vi "rs3 init devices_and_sensors.vi"(6 "rscontext":u64=1752067024, 8 "error in":errorcluster, 9 "api_version":i32=20710, 10 "Select Device":i32, 11 "Select Sensor":i32) -> (0 "error out":errorcluster, 1 "Adv. enable?":i32, 2 "init results":T3, 3 "init error":string, 4 "All Devices":T2(array[cluster]), 5 "Sensor Array":T1(array[cluster]), 7 "Found RealSense":bool)   [LabVIEW 2019, in "libRealSense3.lvlib"]
doc: "Initialized the RealSense device. \nSelect the specific DEVICE and its specific SENSOR. \n\n\nINPUT:\nSelect Device The INDEX to the specific DEVICE handle\nSelect Sensor The INDEX to the specific SENSOR that is part of the selected DEVICE.\n \nOUTPUT:\ninit result Contains all the information about the selected device and its sensor. You will need to use the Dev Out HANDLE to communicate with the device. \n \nselected sensor array Contains the arrays of SENSORS attached to a specific DEVICE.\nall devices Contains array of all device that are attached to the PC."
uses:
  libRealSense3.lvlib
panel:
  # "RS3 Init Device and Sensors"
  # "(C) Intel Corp. 2017,  AGJ"
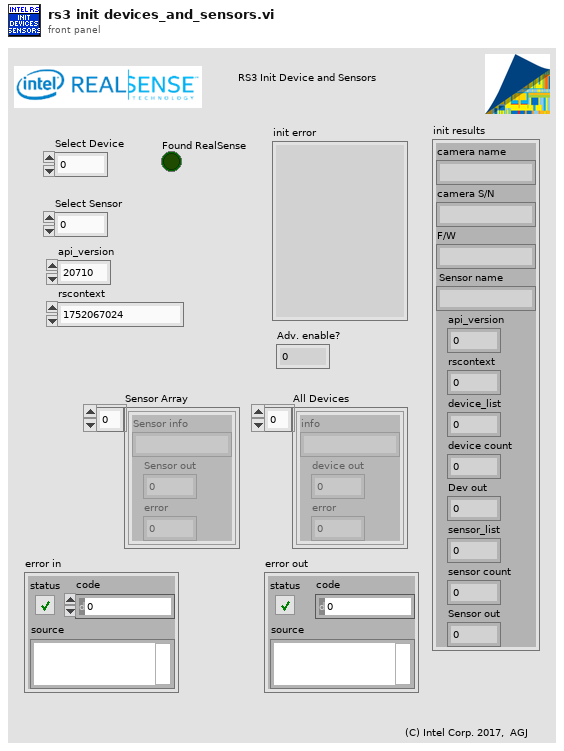
[diagram p1: front panel]
types:
  T1 = cluster{"Sensor info":string, "Sensor out":u64, "error":u64}[]
  T2 = cluster{"info":string, "device out":u64, "error":u64}[]
  T3 = cluster{"camera name":string, "camera S/N":string, "F/W":string, "Sensor name":string, "api_version":i32, "rscontext":u64, "device_list":u64, "device count":i32, "Dev out":u64, "sensor_list":u64, "sensor count":i32, "Sensor out":u64}
  T4 = cluster{"info":string, "device out":u64, "error":u64}
  T5 = cluster{"info":string, "info":string, "info":string, "Sensor info":string, "api_version":i32, "rscontext":u64, "device_list":u64, "device count":i32, "device out":u64, "sensor_list":u64, "sensor count":i32, "Sensor out":u64}
  T6 = cluster{"Sensor info":string, "Sensor out":u64, "error":u64}
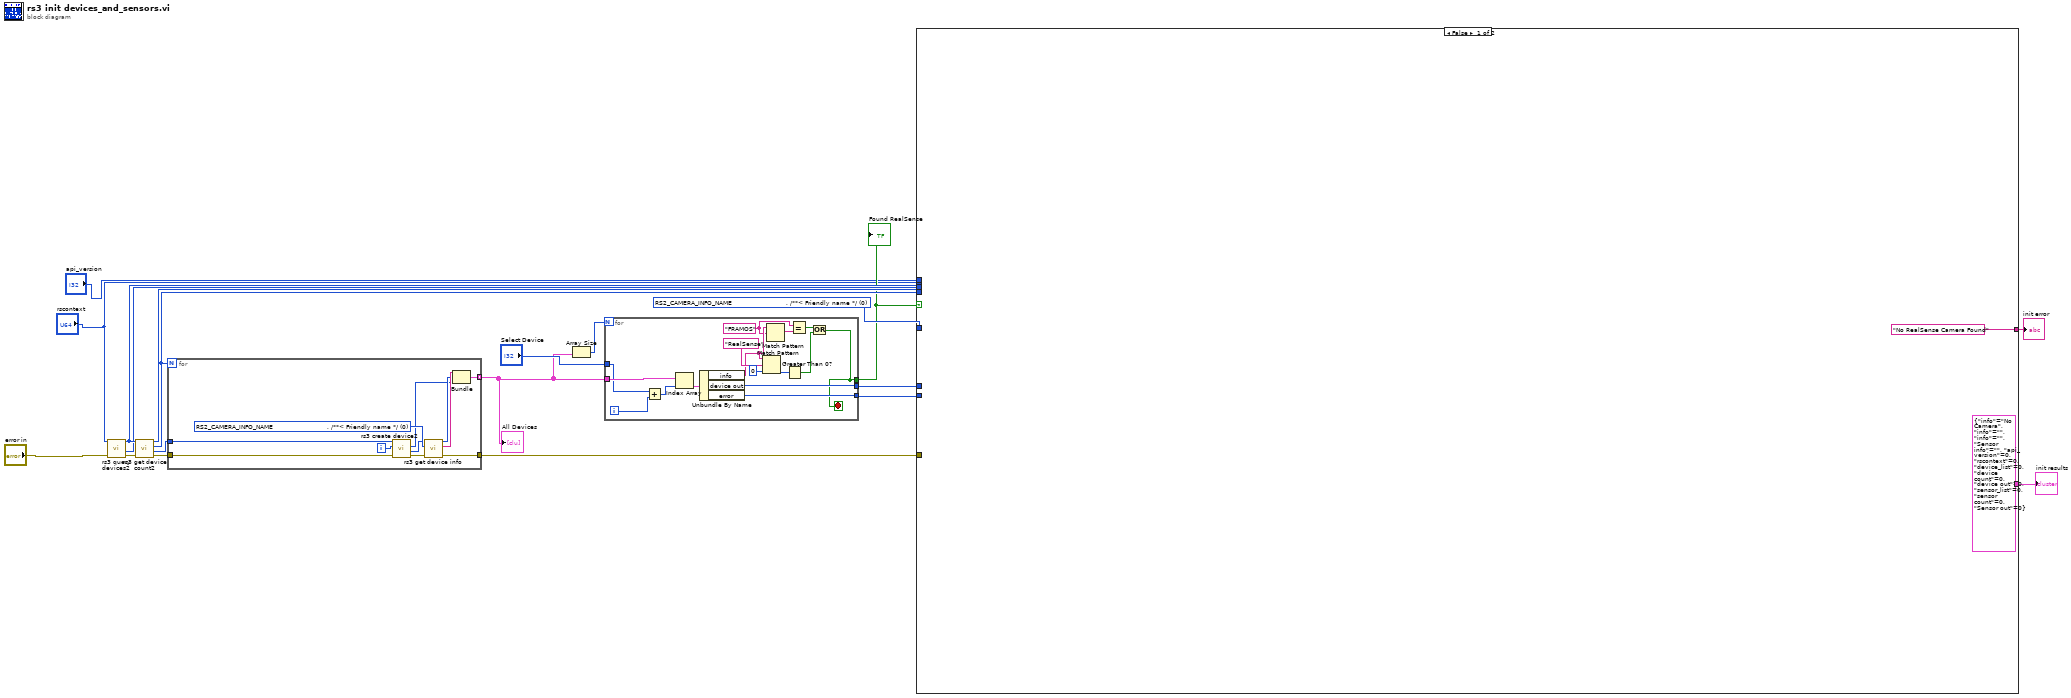
[diagram p0: block diagram]
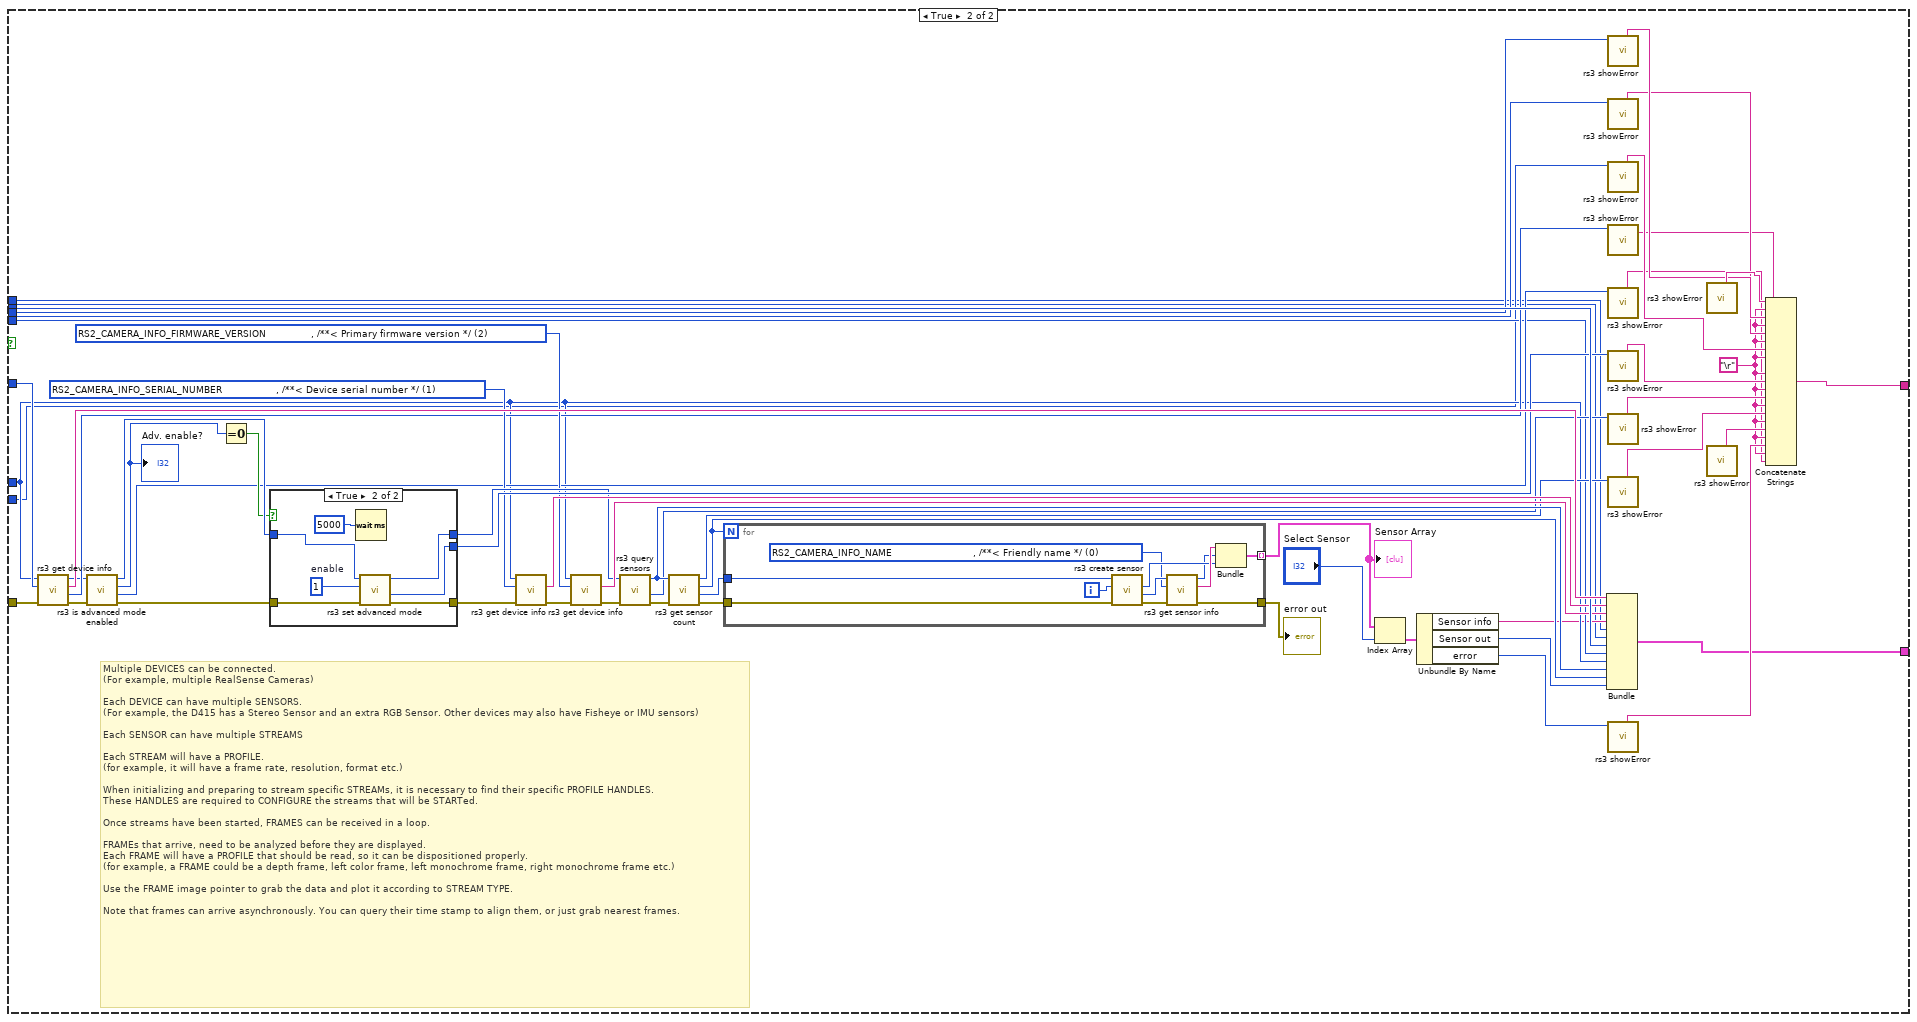
[diagram p2: hidden frame]
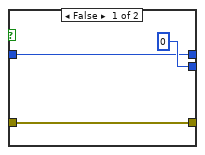
[diagram p3: hidden frame]
diagram:
  w19 = u16 0 items=["    RS2_CAMERA_INFO_NAME                           , /**< Friendly name */", "    RS2_CAMERA_INFO_SERIAL_NUMBER                  , /**< Device serial number */", "    RS2_CAMERA_INFO_FIRMWARE_VERSION               , /**< Primary firmware version */", "    RS2_CAMERA_INFO_PHYSICAL_PORT                       , /**< Unique identifier of the port the device is connected to (platform specific) */", "    RS2_CAMERA_INFO_DEBUG_OP_CODE                  , /**< If device supports firmware logging, this is the command to send to get logs from firmware */", "    RS2_CAMERA_INFO_ADVANCED_MODE                  , /**< True iff the device is in advanced mode */", "    RS2_CAMERA_INFO_PRODUCT_ID                     , /**< Product ID as reported in the USB descriptor */", "    RS2_CAMERA_INFO_CAMERA_LOCKED                  , /**< True iff EEPROM is locked */", "    RS2_CAMERA_INFO_COUNT                            /**< Number of enumeration values. Not a valid input: intended to be used in for-loops. */"] ("RS Camera info")
  n1 = call "rs3 query devices2.vi"("error in (no error)"="error in", "rscontext"="rscontext") -> ("error out"=w17:errorcluster, "error"=w16:u64, "device_list"=w20:u64)  [unwired: 7 in]
  n2 = call "rs3 get device count2.vi"("error in"=w17, "device_list"=w20) -> ("error out"=w11:errorcluster, "device_list_out"=w14:u64, "device count"=w15:i32, "error"=w18:u64)  [unwired: 6 in]
  n3 = for {
    N: w15 -> [_]
    tunnel: w14 -> [w31]
    tunnel: [w25] -> w4 mode=indexing
    tunnel: w11 -> [w24]
    tunnel: [w23] -> w10
    i -> [w30]
    w28 = u16 0 items=["    RS2_CAMERA_INFO_NAME                           , /**< Friendly name */", "    RS2_CAMERA_INFO_SERIAL_NUMBER                  , /**< Device serial number */", "    RS2_CAMERA_INFO_FIRMWARE_VERSION               , /**< Primary firmware version */", "    RS2_CAMERA_INFO_PHYSICAL_PORT                       , /**< Unique identifier of the port the device is connected to (platform specific) */", "    RS2_CAMERA_INFO_DEBUG_OP_CODE                  , /**< If device supports firmware logging, this is the command to send to get logs from firmware */", "    RS2_CAMERA_INFO_ADVANCED_MODE                  , /**< True iff the device is in advanced mode */", "    RS2_CAMERA_INFO_PRODUCT_ID                     , /**< Product ID as reported in the USB descriptor */", "    RS2_CAMERA_INFO_CAMERA_LOCKED                  , /**< True iff EEPROM is locked */", "    RS2_CAMERA_INFO_COUNT                            /**< Number of enumeration values. Not a valid input: intended to be used in for-loops. */"] ("RS Camera info")
    n4 = call "rs3 create device2.vi"("error in (no error)"=w24, "Device index"=w30, "device list in"=w31) -> ("error out"=w29:errorcluster, "Dev out"=w22:u64, "error"=w21:u64)  [unwired: 5 in, 1 out]
    n5 = call "rs3 get device info.vi"("error in (no error)"=w29, "RS Camera info"=w28, "device in"=w22) -> ("error out"=w23:errorcluster, "info"=w27:string, "device out"=w26:u64)  [unwired: 5 in, 1 out]
    n6 = Bundle("info"=w27, "device out"=w26, "error"=w21) -> (w25:T4)  [unwired: 1 in]
  }
  "All Devices" <- w4
  n7 = Array Size(array=w4) -> (size(s)=w5:i32)
  n8 = for {
    N: w5 -> [_]
    tunnel: w4 -> [w47]
    tunnel: "Select Device" -> [w39]
    tunnel: [w45] -> w12
    tunnel: [w44] -> w9
    tunnel: [w33] -> w8
    i -> [w40]
    stop <- w33 stop-if-true
    w35 = "FRAMOS"
    n9 = Add(x=w39, y=w40) -> (x+y=w41:i32)
    n10 = Index Array(array=w47, index=w41) -> (element=w46:T4)
    n11 = Unbundle By Name(w46) -> ("info"=w37:string, "device out"=w45:u64, "error"=w44:u64)
    n12 = Match Pattern(string=w37, regular expression="RealSense" ("string"), offset (0)=0) -> (offset past match=w38:i32)  [unwired: 3 out]
    n13 = Match Pattern(string=w37, regular expression=w35) -> (match substring=w36:string)  [unwired: 1 in, 3 out]
    n14 = Greater Than 0?(x=w38) -> (x > 0?=w32:bool)
    n15 = Equal?(x=w35, y=w36) -> (x = y?=w34:bool)
    n16 = Or(x=w34, y=w32) -> (x .or. y?=w33:bool)
  }
  "Found RealSense" <- w8
  n17 = case shown="False" w8 {
    tunnel: w20 -> [_ w103]
    tunnel: w19 -> [_ w90]
    tunnel: w18 -> [_ w88]
    tunnel: w16 -> [_ w87]
    tunnel: w15 -> [_ w67]
    tunnel: w12 -> [_ w66]
    tunnel: w10 -> [_ w65]
    tunnel: w9 -> [_ w64]
    tunnel: "rscontext" -> [_ w53]
    tunnel: "api_version" -> [_ w52]
    tunnel: ["No RealSense Camera Found" w51] -> w7
    tunnel: [T5 {"info"="No Camera", "info"="", "info"="", "Sensor info"="", "api_version"=0, "rscontext"=0, "device_list"=0, "device count"=0, "device out"=0, "sensor_list"=0, "sensor count"=0, "Sensor out"=0} w50] -> w6
    frame False {
    }
    frame True {
      w69 = "\r"
      w97 = u16 2 items=["    RS2_CAMERA_INFO_NAME                           , /**< Friendly name */", "    RS2_CAMERA_INFO_SERIAL_NUMBER                  , /**< Device serial number */", "    RS2_CAMERA_INFO_FIRMWARE_VERSION               , /**< Primary firmware version */", "    RS2_CAMERA_INFO_PHYSICAL_PORT                       , /**< Unique identifier of the port the device is connected to (platform specific) */", "    RS2_CAMERA_INFO_DEBUG_OP_CODE                  , /**< If device supports firmware logging, this is the command to send to get logs from firmware */", "    RS2_CAMERA_INFO_ADVANCED_MODE                  , /**< True iff the device is in advanced mode */", "    RS2_CAMERA_INFO_PRODUCT_ID                     , /**< Product ID as reported in the USB descriptor */", "    RS2_CAMERA_INFO_CAMERA_LOCKED                  , /**< True iff EEPROM is locked */", "    RS2_CAMERA_INFO_COUNT                            /**< Number of enumeration values. Not a valid input: intended to be used in for-loops. */"] ("RS Camera info")
      w96 = u16 1 items=["    RS2_CAMERA_INFO_NAME                           , /**< Friendly name */", "    RS2_CAMERA_INFO_SERIAL_NUMBER                  , /**< Device serial number */", "    RS2_CAMERA_INFO_FIRMWARE_VERSION               , /**< Primary firmware version */", "    RS2_CAMERA_INFO_PHYSICAL_PORT                       , /**< Unique identifier of the port the device is connected to (platform specific) */", "    RS2_CAMERA_INFO_DEBUG_OP_CODE                  , /**< If device supports firmware logging, this is the command to send to get logs from firmware */", "    RS2_CAMERA_INFO_ADVANCED_MODE                  , /**< True iff the device is in advanced mode */", "    RS2_CAMERA_INFO_PRODUCT_ID                     , /**< Product ID as reported in the USB descriptor */", "    RS2_CAMERA_INFO_CAMERA_LOCKED                  , /**< True iff EEPROM is locked */", "    RS2_CAMERA_INFO_COUNT                            /**< Number of enumeration values. Not a valid input: intended to be used in for-loops. */"] ("RS Camera info")
      # "Multiple DEVICES can be connected. \n(For example, multiple RealSense Cameras)\n\nEach DEVICE can have multiple SENSORS. \n(For example, the D415 has a Stereo Sensor and an extra RGB Sensor. Other devices may also have Fisheye or IMU sensors) \n\nEach SENSOR can have multiple STREAMS\n\nEach STREAM will have a PROFILE. \n(for example, it will have a frame rate, resolution, format etc.)\n\nWhen initializing and preparing to stream specific STREAMs, it is necessary to find their specific PROFILE HANDLES.\nThese HANDLES are required to CONFIGURE the streams that will be STARTed. \n\nOnce streams have been started, FRAMES can be received in a loop. \n \nFRAMEs that arrive, need to be analyzed before they are displayed. \nEach FRAME will have a PROFILE that should be read, so it can be dispositioned properly.\n(for example, a FRAME could be a depth frame, left color frame, left monochrome frame, right monochrome frame etc.)\n\nUse the FRAME image pointer to grab the data and plot it according to STREAM TYPE.\n\nNote that frames can arrive asynchronously. You can query their time stamp to align them, or just grab nearest frames."
      n18 = call "rs3 get device info.vi"("error in (no error)"=w65, "RS Camera info"=w90, "device in"=w66) -> ("error out"=w76:errorcluster, "error"=w89:u64, "info"=w104:string, "device out"=w74:u64)  [unwired: 5 in]
      n19 = call "rs3 is advanced mode enabled.vi"("error in (no error)"=w76, "device in"=w74) -> ("error out"=w75:errorcluster, "error"=w70:u64, "enable?"=w72:i32, "device out"=w73:u64)  [unwired: 6 in]
      "Adv. enable?" <- w72
      n20 = Equal To 0?(x=w72) -> (x = 0?=w71:bool)
      n21 = case shown="True" w71 {
        tunnel: [u64 0 ("error") w126] -> w100
        tunnel: [w117 w124] -> w99
        tunnel: w73 -> [w117 w123]
        tunnel: [w119 w122] -> w98
        tunnel: w75 -> [w119 w121]
        frame False {
        }
        frame True {
          w125 = 1  # enable
          n22 = Wait (ms)(milliseconds to wait=u32 5000) -> ()  [unwired: 1 out]
          n23 = call "rs3 set advanced mode.vi"("error in (no error)"=w121, "enable"=w125, "device in"=w123) -> ("error out"=w122:errorcluster, "error"=w126:u64, "device out"=w124:u64)  [unwired: 6 in]
        }
      }
      n24 = call "rs3 get device info.vi"("error in (no error)"=w98, "RS Camera info"=w96, "device in"=w66) -> ("error out"=w94:errorcluster, "info"=w101:string)  [unwired: 5 in, 2 out]
      n25 = call "rs3 get device info.vi"("error in (no error)"=w94, "RS Camera info"=w97, "device in"=w66) -> ("error out"=w95:errorcluster, "info"=w102:string)  [unwired: 5 in, 2 out]
      n26 = call "rs3 query sensors.vi"("error in (no error)"=w95, "device in"=w99) -> ("error out"=w92:errorcluster, "error"=w91:u64, "sensor_list"=w105:u64)  [unwired: 7 in]
      n27 = call "rs3 get sensor count.vi"("error in"=w92, "sensor_list"=w105) -> ("error out"=w62:errorcluster, "sensor_list_out"=w61:u64, "sensor count"=w63:i32, "error"=w93:u64)  [unwired: 6 in]
      n28 = for {
        N: w63 -> [_]
        tunnel: w62 -> [w116]
        tunnel: w61 -> [w113]
        tunnel: [w107] -> w60 mode=indexing
        tunnel: [w106] -> w55
        i -> [w114]
        w109 = u16 0 items=["    RS2_CAMERA_INFO_NAME                           , /**< Friendly name */", "    RS2_CAMERA_INFO_SERIAL_NUMBER                  , /**< Device serial number */", "    RS2_CAMERA_INFO_FIRMWARE_VERSION               , /**< Primary firmware version */", "    RS2_CAMERA_INFO_PHYSICAL_PORT                       , /**< Unique identifier of the port the device is connected to (platform specific) */", "    RS2_CAMERA_INFO_DEBUG_OP_CODE                  , /**< If device supports firmware logging, this is the command to send to get logs from firmware */", "    RS2_CAMERA_INFO_ADVANCED_MODE                  , /**< True iff the device is in advanced mode */", "    RS2_CAMERA_INFO_PRODUCT_ID                     , /**< Product ID as reported in the USB descriptor */", "    RS2_CAMERA_INFO_CAMERA_LOCKED                  , /**< True iff EEPROM is locked */", "    RS2_CAMERA_INFO_COUNT                            /**< Number of enumeration values. Not a valid input: intended to be used in for-loops. */"] ("RS Sensor info")
        n29 = call "rs3 create sensor.vi"("error in (no error)"=w116, "Sensor index"=w114, "Sensor list"=w113) -> ("error out"=w115:errorcluster, "Sensor out"=w111:u64, "error"=w110:u64)  [unwired: 5 in, 1 out]
        n30 = call "rs3 get sensor info.vi"("error in (no error)"=w115, "RS Camera info"=w109, "Sensor in"=w111) -> ("error out"=w106:errorcluster, "Sensor info"=w112:string, "Sensor out"=w108:u64)  [unwired: 5 in, 1 out]
        n31 = Bundle("Sensor info"=w112, "Sensor out"=w108, "error"=w110) -> (w107:T6)  [unwired: 1 in]
      }
      "error out" <- w55
      "Sensor Array" <- w60
      n32 = Index Array(array=w60, index="Select Sensor") -> (element=w58:T6)
      n33 = Unbundle By Name(w58) -> ("Sensor info"=w54:string, "Sensor out"=w57:u64, "error"=w56:u64)
      n34 = Bundle("info"=w104, "info"=w101, "info"=w102, "Sensor info"=w54, "api_version"=w52, "rscontext"=w53, "device_list"=w103, "device count"=w67, "device out"=w66, "sensor_list"=w105, "sensor count"=w63, "Sensor out"=w57) -> (w50:T5)  [unwired: 1 in]
      n35 = call "rs3 showError.vi"("error"=w87) -> ("Error summary"=w85:string)  [unwired: 6 in, 4 out]
      n36 = call "rs3 showError.vi"("error"=w88) -> ("Error summary"=w84:string)  [unwired: 6 in, 4 out]
      n37 = call "rs3 showError.vi"("error"=w64) -> ("Error summary"=w83:string)  [unwired: 6 in, 4 out]
      n38 = call "rs3 showError.vi"("error"=w89) -> ("Error summary"=w82:string)  [unwired: 6 in, 4 out]
      n39 = call "rs3 showError.vi"("error"=w70) -> ("Error summary"=w68:string)  [unwired: 6 in, 4 out]
      n40 = call "rs3 showError.vi"("error"=w100) -> ("Error summary"=w81:string)  [unwired: 6 in, 4 out]
      n41 = call "rs3 showError.vi"("error"=w91) -> ("Error summary"=w80:string)  [unwired: 6 in, 4 out]
      n42 = call "rs3 showError.vi"("error"=w93) -> ("Error summary"=w79:string)  [unwired: 6 in, 4 out]
      n43 = call "rs3 showError.vi"("error"=w56) -> ("Error summary"=w77:string)  [unwired: 6 in, 4 out]
      n44 = call "rs3 showError.vi"() -> ("Error summary"=w86:string)  [unwired: 7 in, 4 out]
      n45 = call "rs3 showError.vi"() -> ("Error summary"=w78:string)  [unwired: 7 in, 4 out]
      n46 = Concatenate Strings(w86, w69, w85, w69, w84, w69, w83, w69, w82, w69, w81, w69, w80, w69, w79, w69, w78, w69, w77, w69, w68) -> (w51:string)
    }
  }
  "init error" <- w7
  "init results" <- w6
